vi "Process.vi"(8 "error in":errorcluster, 11 "Inst UI.AH2500":refnum<class "Inst UI.AH2500.lvclass">) -> (0 "error out":errorcluster, 3 "Inst UI.AH2500 out":refnum<class "Inst UI.AH2500.lvclass">)   [LabVIEW 2019, in "Inst UI.AH2500.lvclass"]
doc: "---------------------------------------------------------------\nJKI State Machine Objects™\nhttp://jki.net/state-machine-objects/\nCopyright (C) 2005-2015, JKI <info@jki.net>\nALL RIGHTS RESERVEDJKI State Machine Objects (SMO) 1.0.0.5\nJKI - JKI\nCopyright (c) 2016, JKI"
uses:
  Inst UI.AH2500.lvclass
  C:/Program Files (x86)/National Instruments/LabVIEW 2019/vi.lib/JKI/JKI SMO/SMO/SMO.lvclass
  C:/Program Files (x86)/National Instruments/LabVIEW 2019/user.lib/LevyLab/Instrument Framework/SMOs/Instrument UI/Instrument UI.lvclass
  C:/Program Files (x86)/National Instruments/LabVIEW 2019/vi.lib/JKI/JKI SMO/SMO.UI/SMO.UI.lvclass
  Inst.AH2500/Typedefs/Inst.AH2500.getAll--Cluster.ctl
  Inst.AH2500/Inst.AH2500.lvclass
  C:/Program Files (x86)/National Instruments/LabVIEW 2019/user.lib/LevyLab/Instrument Framework/SMOs/Instrument/Instrument.lvclass
  Inst UI.AH2500.UI--Cluster.ctl
  Inst.AH2500/Typedefs/Inst.AH2500.Configuration--Cluster.ctl
  <userlib>/LevyLab/Instrument Framework/SMOs/Configuration/Configuration.lvclass
  <userlib>/LevyLab/Instrument Framework/SMOs/RemoteControl/Typedefs/Message--Cluster.ctl
  <userlib>/LevyLab/Instrument Framework/SMOs/Instrument UI/Instrument UI.lvclass/Instrument UI.ctl
  Inst.AH2500/Inst.AH2500.lvclass/Inst.AH2500.ctl
  <vilib>/JKI/JKI SMO/SMO/SMO.lvclass/SMO.ctl
  <userlib>/LevyLab/Instrument Framework/SMOs/Configuration/Configuration.lvclass/Configuration.ctl
  <userlib>/LevyLab/Instrument Framework/SMOs/Instrument/Instrument.lvclass/Instrument.ctl
  <userlib>/LevyLab/Instrument Framework/SMOs/Instrument/Typedefs/Client Type--Enum.ctl
  09e9697b-516c-49fb-b2dc-692589121b6f.vi
  <vilib>/JKI/JKI SMO/SMO/Private/ReftoDVR--SMO.vi
  09e9697b-516c-49fb-b2dc-692589121b6f.vi/e95de145-570b-4452-909a-60166876b235.vi
  09e9697b-516c-49fb-b2dc-692589121b6f.vi/e95de145-570b-4452-909a-60166876b235.vi/36141e6f-c45c-4e10-a95a-9d5fe44f6ec9.vi
  <userlib>/LevyLab/Instrument Framework/SMOs/Instrument/API/Send and Receive.vi
  09e9697b-516c-49fb-b2dc-692589121b6f.vi/e95de145-570b-4452-909a-60166876b235.vi/d03f3c8e-ad6b-4901-9eeb-1b6090619d7a.vi
  <userlib>/LevyLab/Instrument Framework/SMOs/Instrument/Private/Get Client Type.vi
  09e9697b-516c-49fb-b2dc-692589121b6f.vi/e95de145-570b-4452-909a-60166876b235.vi/36141e6f-c45c-4e10-a95a-9d5fe44f6ec9.vi/1de991dd-cae7-4693-a0cb-9204aa9fd824.vi
  09e9697b-516c-49fb-b2dc-692589121b6f.vi/e95de145-570b-4452-909a-60166876b235.vi/36141e6f-c45c-4e10-a95a-9d5fe44f6ec9.vi/fe17b767-a917-482f-9198-46e18cb5e30b.vi
  09e9697b-516c-49fb-b2dc-692589121b6f.vi/e95de145-570b-4452-909a-60166876b235.vi/d03f3c8e-ad6b-4901-9eeb-1b6090619d7a.vi/65f50c0c-55d1-4f0e-9c2f-0837c701ede4.vi
  09e9697b-516c-49fb-b2dc-692589121b6f.vi/e95de145-570b-4452-909a-60166876b235.vi/d03f3c8e-ad6b-4901-9eeb-1b6090619d7a.vi/7c5fe90f-b0b4-4563-867a-64d0d40b5a7e.vi
  09e9697b-516c-49fb-b2dc-692589121b6f.vi/e95de145-570b-4452-909a-60166876b235.vi/d03f3c8e-ad6b-4901-9eeb-1b6090619d7a.vi/65f50c0c-55d1-4f0e-9c2f-0837c701ede4.vi/ad86d9d7-fa14-4d0e-9eae-53db6c5c549a.vi
  09e9697b-516c-49fb-b2dc-692589121b6f.vi/e95de145-570b-4452-909a-60166876b235.vi/d03f3c8e-ad6b-4901-9eeb-1b6090619d7a.vi/65f50c0c-55d1-4f0e-9c2f-0837c701ede4.vi/f29f3462-655b-41ba-8fda-c1e4ae9d02a0.vi
  <userlib>/LevyLab/Instrument Framework/SMOs/Instrument/Private/Get RC Connection Status.vi
  <userlib>/LevyLab/Instrument Framework/SMOs/Instrument/API/Enum to String.vi
  <userlib>/LevyLab/Instrument Framework/SMOs/RemoteControl/API/Send and Receive.vi
  <vilib>/Utility/Data Type/Get Type Information.vi
  <vilib>/JDP Science/JSONtext/JSON text to Variant.vi
  <vilib>/JDP Science/JSONtext/Variant to JSON Text.vi
  <vilib>/National Instruments/GUID Generator/Guid Generator.vi
  <userlib>/LevyLab/Instrument Framework/SMOs/Instrument/Private/Instrument.MessageFromProcess.EventStructure.vi
  <userlib>/LevyLab/Instrument Framework/SMOs/Instrument/Instrument.lvclass
  <vilib>/JDP Science/JSONtext/LVClass Serializer/JSONtext LVClass Serializer.lvclass
  <userlib>/LevyLab/Instrument Framework/SMOs/Instrument UI/Instrument UI.lvclass
  <vilib>/JKI/JKI SMO/SMO/SMO.lvclass
  <vilib>/JKI/JKI SMO/SMO.UI/SMO.UI.lvclass
  <userlib>/LevyLab/Instrument Framework/SMOs/RemoteControl/RemoteControl.lvclass
panel:
  in  "Enable Output 2":bool
  in  "I/O":bool
  out "STUFF":bool
  out "LOSS":string="bridge"
  out "CAPACITANCE - pF":string="cap"
  out "Status":string="SMO State: Stopped"
  out "version":string="vDevelopment"
  # "AH 2500A ULTRA-PRECISION 1kHz CAPACITANCE BRIDGE"
  # "SMO UI Template"
  # "For instructions on how to use the JKI State Machine Objects, examples and video tutorials, visit:\nhttp://jki.net/state-machine-objects/\n\nJKI State Machine Objects™\nhttp://jki.net/state-machine-objects/\nCopyright (C) 2005-2015, JKI <info@jki.net>\nALL RIGHTS RESERVED"
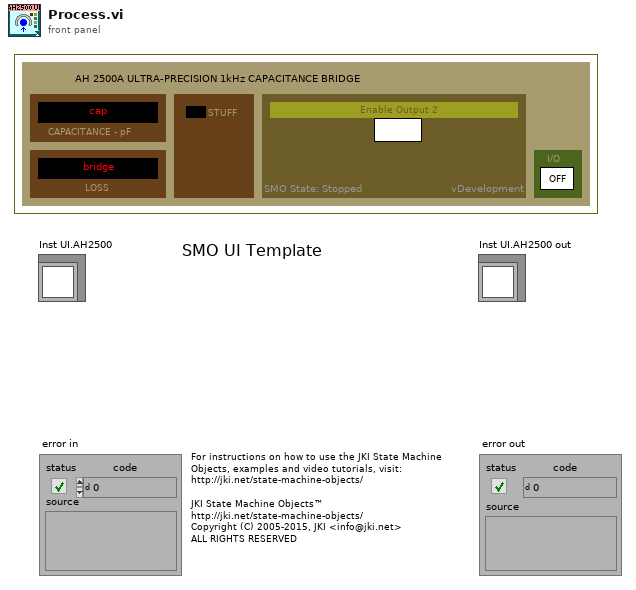
[diagram p1: front panel]
types:
  T1 = enum32{"invalid app kind", "Development System", "Run Time System", "Student Edition", "Embedded LabVIEW", "Evaluation", "Custom"}
  T2 = enum32{"Invalid", "Standard", "Closed", "Hidden", "Minimized", "Maximized"}
  T3 = typedef "Instrument.lvclass/Client Type--Enum.ctl" = enum16{"Remote", "Local"}
  T4 = typedef "RemoteControl.lvclass/Message--Cluster.ctl" = cluster{"Command":string, "Data":variant, "ID":string}
  T5 = typedef "Inst.AH2500.lvclass/Inst.AH2500.Configuration--Cluster.ctl" = cluster{"Example Setting 1":dbl, "Example Setting 2":dbl, "Example Setting 3":string}
  T6 = typedef "Inst.AH2500.lvclass/Inst.AH2500.getAll--Cluster.ctl" = cluster{"capacitance (pF)":dbl, "loss (nS)":dbl, "Vexc (V)":dbl}
  T7 = typedef "Inst UI.AH2500.lvclass/Inst UI.AH2500.UI--Cluster.ctl" = cluster{"Ch1 (V)":dbl, "Ch2 (V)":dbl, "Slew (V/s)":dbl}
  T8 = cluster{"Core":cluster{"Current VI Reference":refnum<vi>, "Close Panel on Exit?":bool, "Last Error":cluster{"error":errorcluster, "previous state":string, "remaining states":string}, "Shutdown?":bool}, "Instrument UI":refnum<class "Inst UI.AH2500.lvclass">, "Instrument":refnum<class "Inst.AH2500.lvclass">, "Configuration":refnum<class "Configuration.lvclass">, "Config Cluster":T5, "getAll":T6, "UI Cluster":T7, "Message":T4}
  T9 = typedef "SMO.lvclass/SMOState --Enum.ctl" = enum16{"unknown", "Created", "Started", "Stopped"}
  T10 = cluster{"Current VI Reference":refnum<vi>, "Close Panel on Exit?":bool, "Last Error":cluster{"error":errorcluster, "previous state":string, "remaining states":string}, "Shutdown?":bool}
  T11 = typedef "SMO.lvclass/Protected Events.ctl" = cluster{"StopProcesses":refnum<user-event>, "AbortProcesses":refnum<user-event>, "Config Changed":refnum<user-event>, "Dependency":refnum<user-event>}
  T12 = typedef "Instrument.lvclass/PublicEvents--Cluster.ctl" = cluster{"MessageFromProcess":refnum<user-event>}
  T13 = typedef "Inst.AH2500.lvclass/PublicEvents--Cluster.ctl" = cluster{"MessageFromProcess":refnum<user-event>}
  T14 = typedef "SMO.lvclass/Public Events.ctl" = cluster{"Error":refnum<user-event>, "State":refnum<user-event>, "Reserve State":refnum<user-event>}
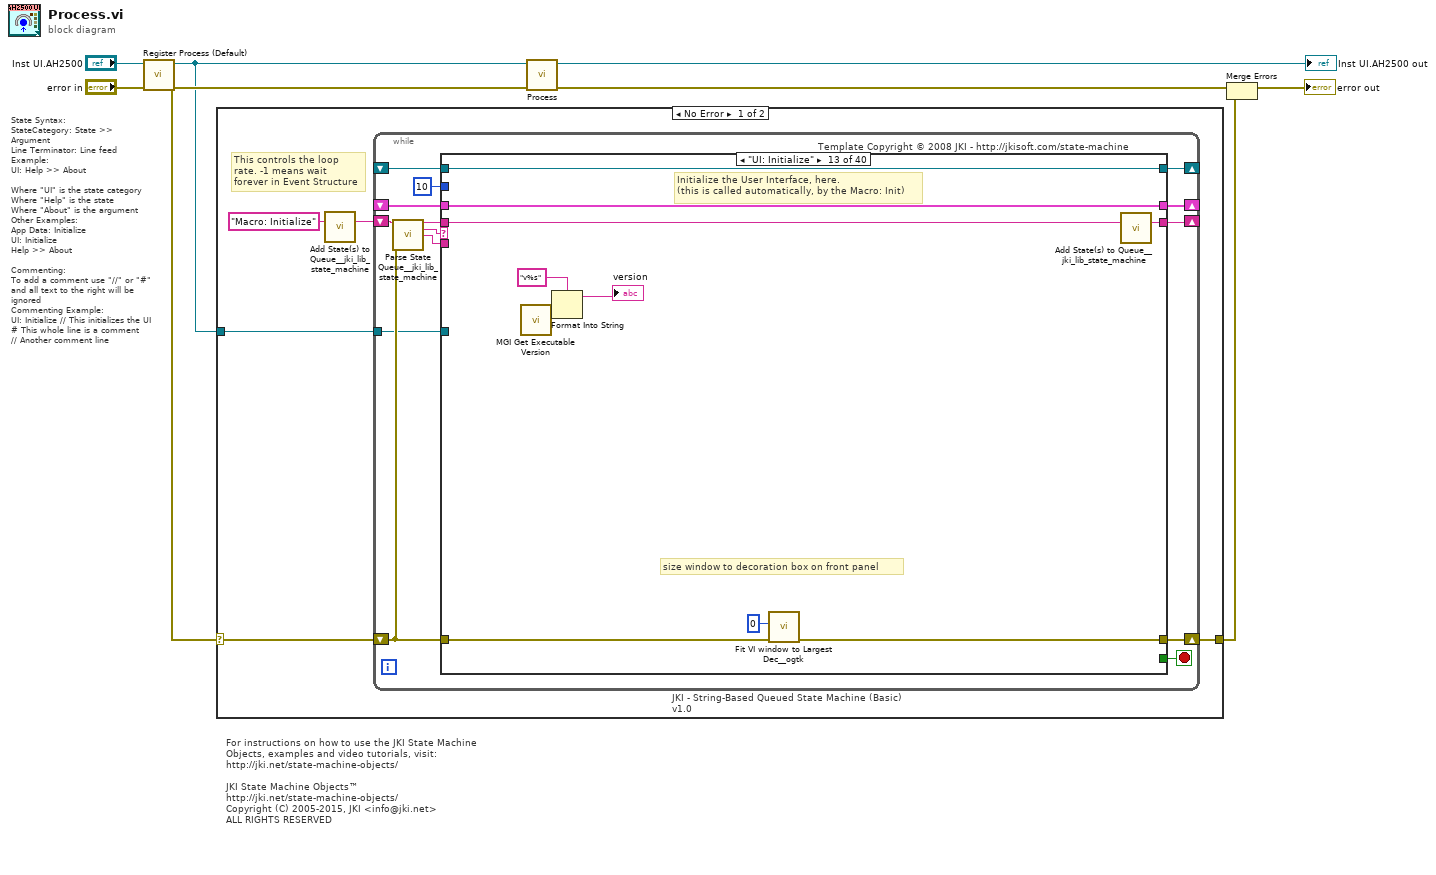
[diagram p0: block diagram]
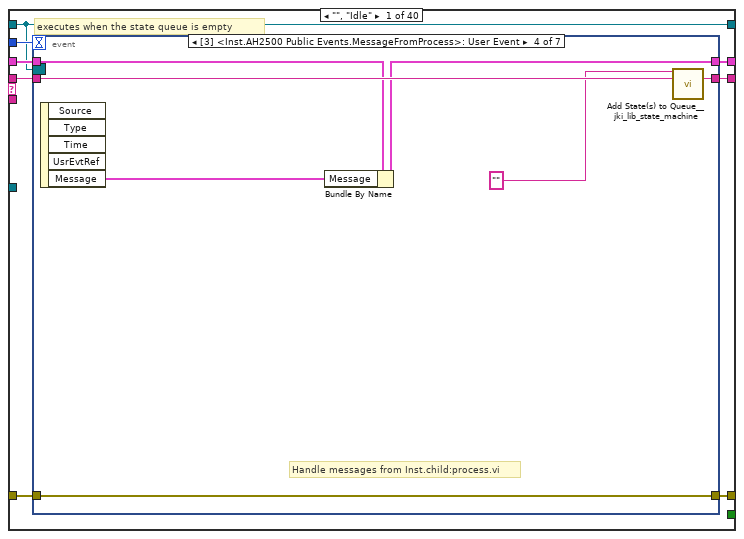
[diagram p2: hidden frame]
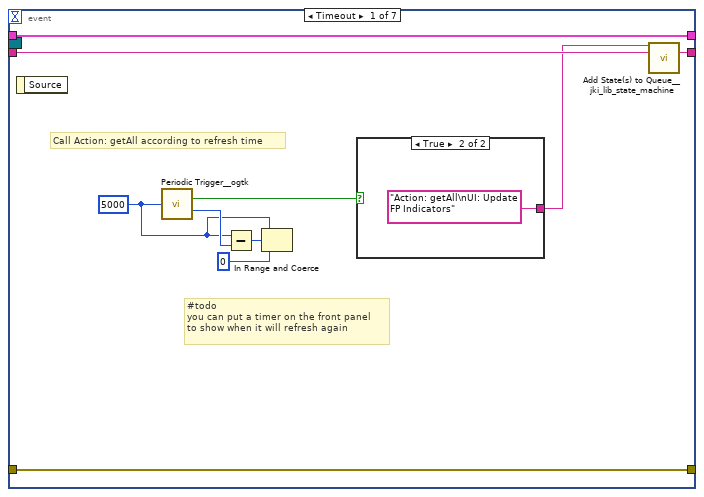
[diagram p3: hidden frame]
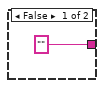
[diagram p4: hidden frame]
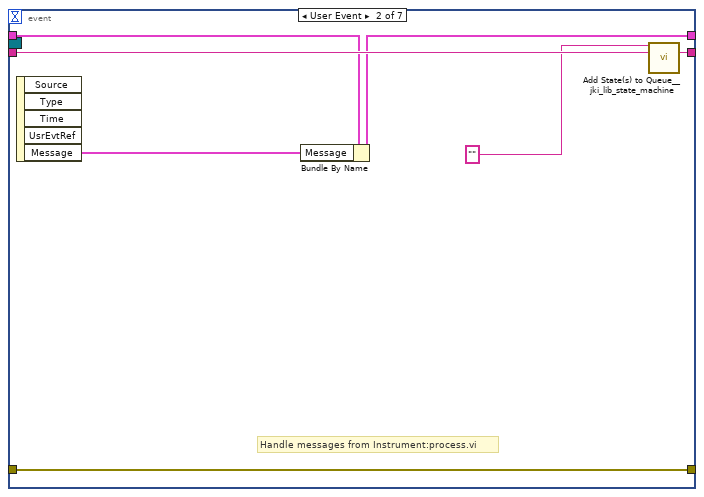
[diagram p5: hidden frame]
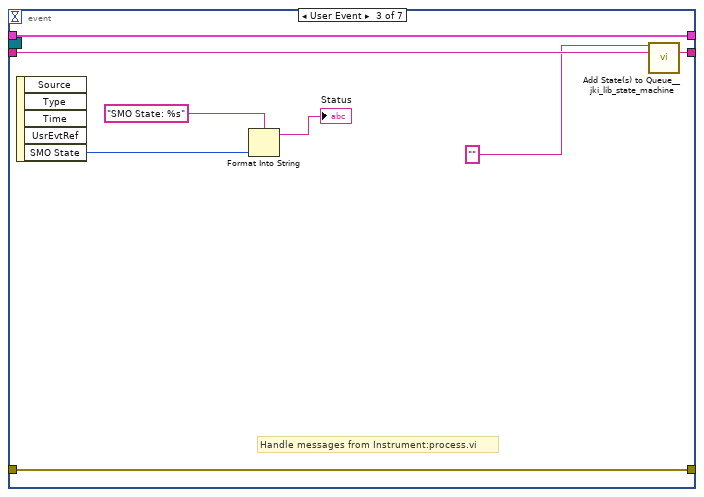
[diagram p6: hidden frame]
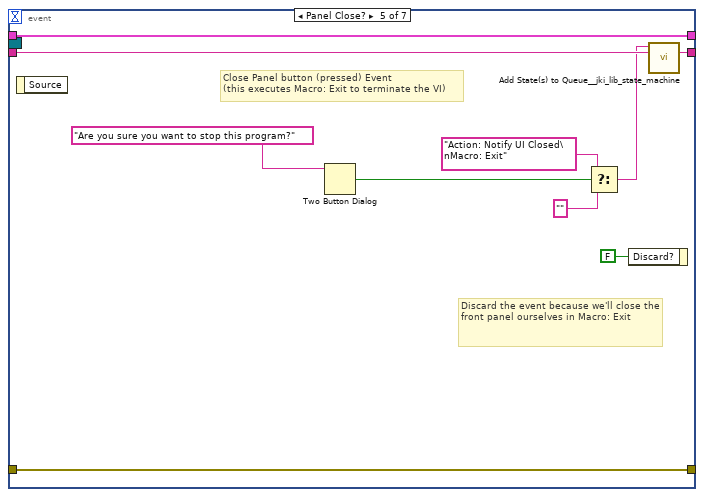
[diagram p7: hidden frame]
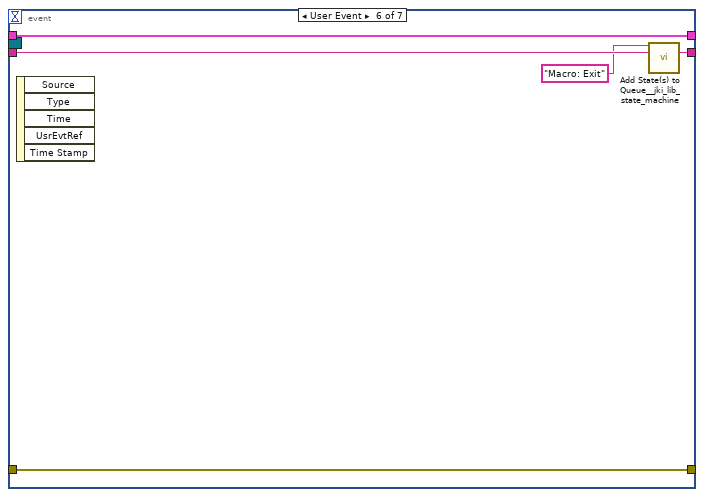
[diagram p8: hidden frame]
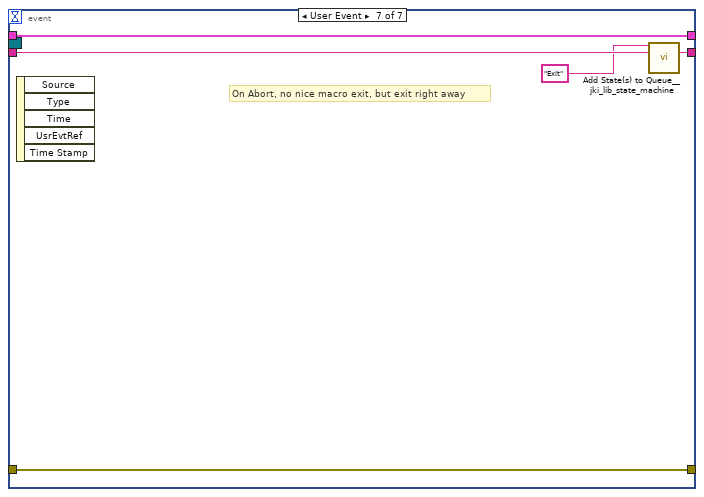
[diagram p9: hidden frame]
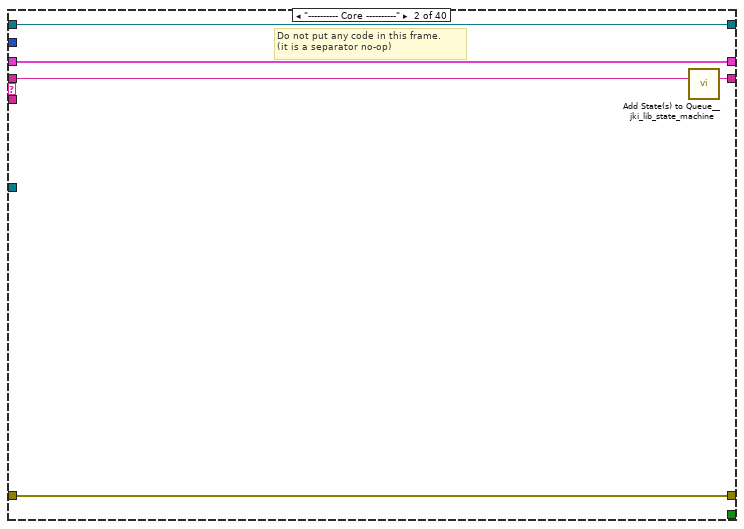
[diagram p10: hidden frame]
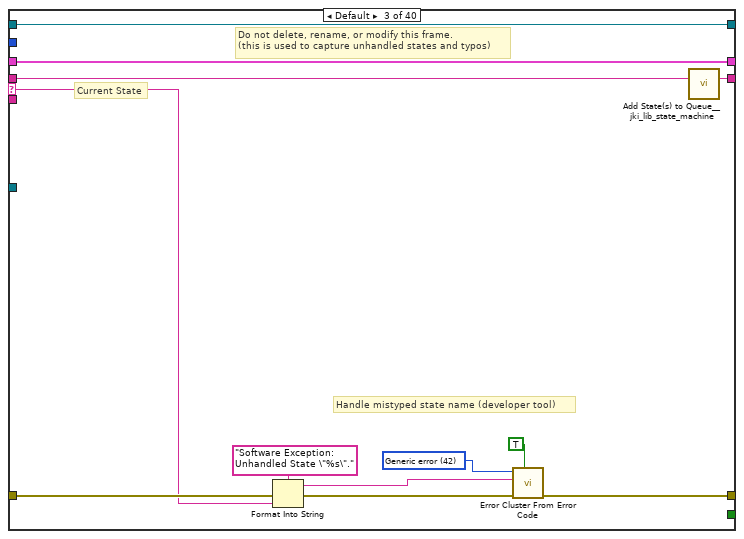
[diagram p11: hidden frame]
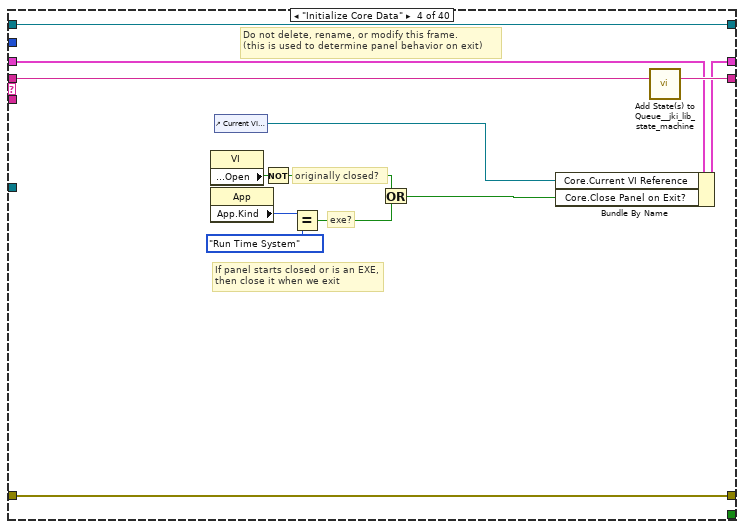
[diagram p12: hidden frame]
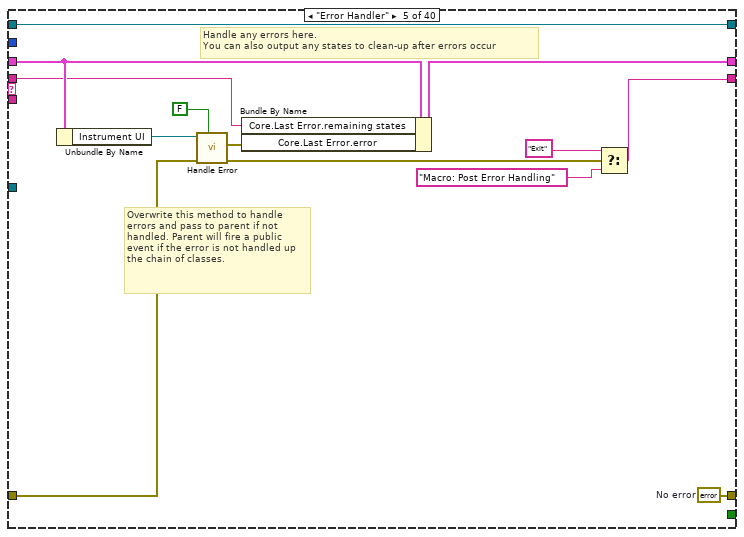
[diagram p13: hidden frame]
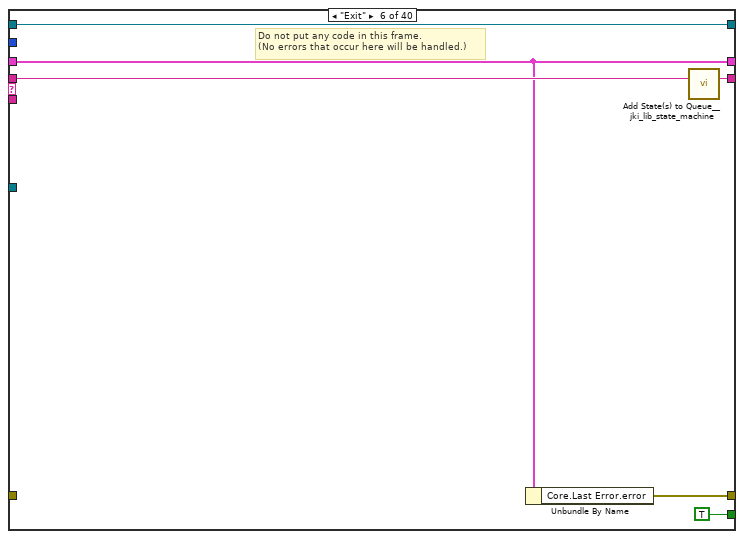
[diagram p14: hidden frame]
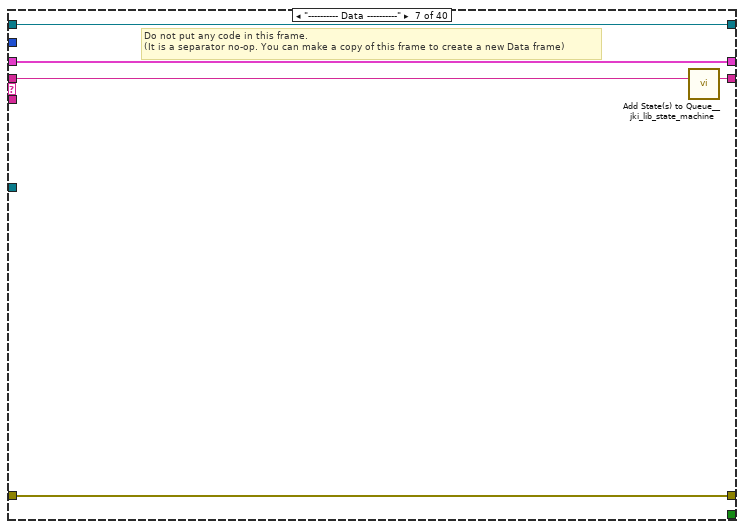
[diagram p15: hidden frame]
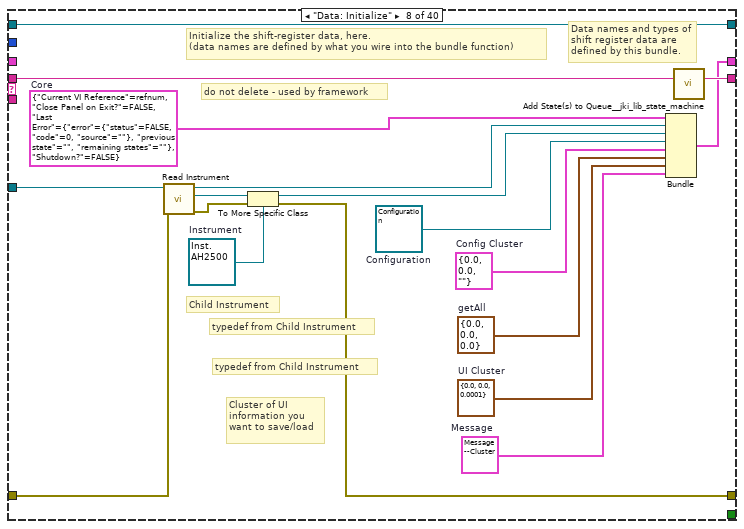
[diagram p16: hidden frame]
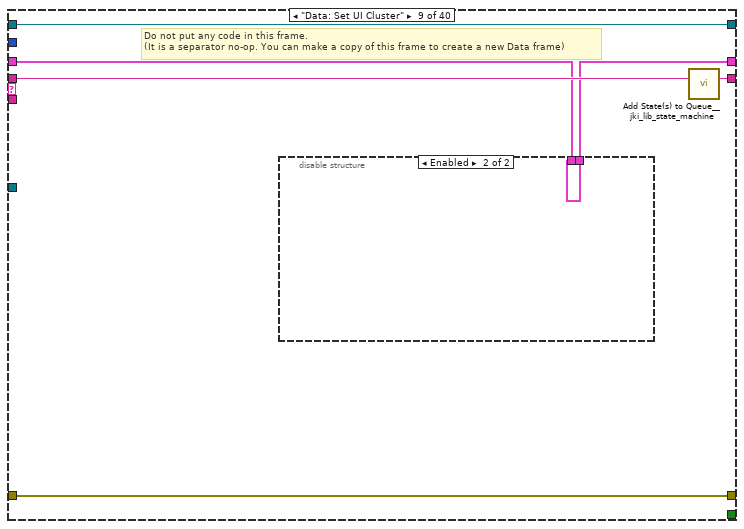
[diagram p17: hidden frame]
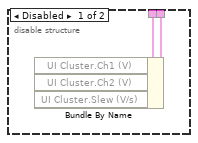
[diagram p18: hidden frame]
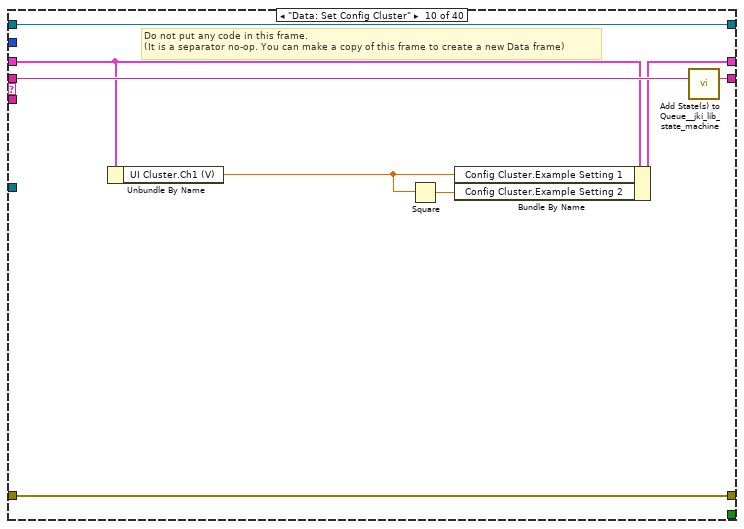
[diagram p19: hidden frame]
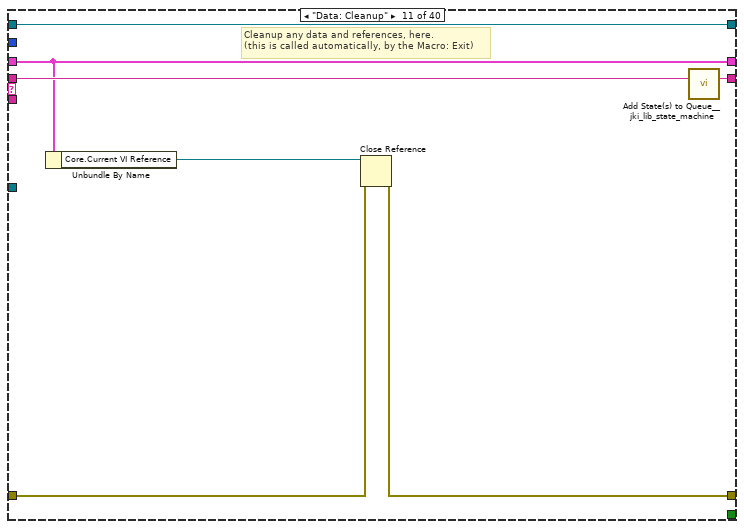
[diagram p20: hidden frame]
diagram:
  # "State Syntax:\nStateCategory: State >> Argument\nLine Terminator: Line feed\nExample:\nUI: Help >> About\n\nWhere \"UI\" is the state category\nWhere \"Help\" is the state\nWhere \"About\" is the argument\nOther Examples:\nApp Data: Initialize\nUI: Initialize\nHelp >> About\n\nCommenting:\nTo add a comment use \"//\" or \"#\" and all text to the right will be ignored\nCommenting Example:\nUI: Initialize // This initializes the UI\n# This whole line is a comment\n// Another comment line"
  # "For instructions on how to use the JKI State Machine Objects, examples and video tutorials, visit:\nhttp://jki.net/state-machine-objects/\n\nJKI State Machine Objects™\nhttp://jki.net/state-machine-objects/\nCopyright (C) 2005-2015, JKI <info@jki.net>\nALL RIGHTS RESERVED"
  n1 = call <vilib>:"Register Process (Default).vi"("error in (no error)"="error in", "SMO"="Inst UI.AH2500") -> ("error out"=w5:errorcluster, "SelfRef"=w4:refnum<class "Inst UI.AH2500.lvclass">)  [unwired: 8 in]
  n2 = case shown="No Error" w5 {
    selector: w5 -> [w10 w487]
    tunnel: w4 -> [w11 _]
    tunnel: [w9 w487] -> w1
    frame No Error {
      # "This controls the loop rate. -1 means wait forever in Event Structure"
      n3 = call <vilib>:"Add State(s) to Queue__jki_lib_state_machine.vi"("State(s) in (\"\")"="Macro: Initialize") -> ("States Out"=w13:string)  [unwired: 14 in]
      n4 = while "JKI - String-Based Queued State Machine (Basic) v1.0" {
        shift-right: [w20] -> _
        shift-left: _ -> [w19]
        shift-right: [w23] -> w9
        shift-left: w10 -> [w17]
        shift-right: [w22] -> _
        shift-left: w13 -> [w24]
        tunnel: w11 -> [w16]
        shift-right: [w15] -> _
        shift-left: _ -> [w14]
        stop <- w21 stop-if-true
        # "Template Copyright © 2008 JKI - http://jkisoft.com/state-machine"
        n5 = call <vilib>:"Parse State Queue__jki_lib_state_machine.vi"("State Queue"=w24, "Error In (no error)"=w17) -> ("Remaining States"=w26:string, "Current State"=w27:string, "Arguments"=w25:string)  [unwired: 11 in]
        n6 = case shown="\"UI: Initialize\"" w27 {
          selector: w27 -> [_ _ w96 _ _ _ _ _ _ _ _ _ _ _ _ _ _ _ _ _ _ _ _ _ _ _ _ _ _ _ _ _ _ _ _ _ _ _ _ _]
          tunnel: w26 -> [w35 w94 w100 w119 w123 w138 w143 w161 w167 w178 w185 w190 w200 w205 w217 w224 w240 w272 w281 w293 w303 w309 w324 w329 w340 w347 w352 w371 w377 w382 w397 w405 w417 w424 w431 w443 w456 w466 w476 w486]
          tunnel: w25 -> [_ _ _ _ _ _ _ _ _ _ _ _ _ _ _ w218 w234 _ _ _ _ _ _ _ _ _ _ _ _ _ _ _ _ _ _ _ _ _ _ _]
          tunnel: w19 -> [w33 w91 w98 w110 w126 w134 w140 _ w163 w174 w179 w187 w198 w201 w213 w222 w236 w269 w277 w283 w300 w306 w311 w326 w337 w342 w349 w369 w375 w379 w390 w402 w408 w419 w425 w435 w450 w458 w471 w481]
          tunnel: [w32 w92 w102 w116 w128 w133 w141 w148 w165 w176 w181 w188 w195 w203 w214 w219 w237 w270 w279 w291 w301 w307 w322 w327 w331 w343 w350 w366 w372 w380 w383 w400 w409 w421 w426 w440 w453 w463 w467 w477] -> w23
          tunnel: w17 -> [w31 w92 w101 w116 w122 _ w141 w145 w165 w176 w182 w188 w196 w203 w214 w220 w238 w270 w279 w291 w301 w307 w322 w327 w332 w344 w350 w356 w373 w380 w392 w398 w410 w421 w427 w436 w445 w459 w468 w478]
          tunnel: [w34 w93 w99 w118 w120 w137 w142 w160 w166 w177 w184 w189 w199 w204 w216 w223 w239 w271 w280 w292 w302 w308 w323 w328 w339 w346 w351 w370 w376 w381 w396 w404 w416 w423 w430 w442 w455 w465 w475 w485] -> w22
          tunnel: [_ _ _ _ _ TRUE _ _ _ _ _ _ _ _ _ _ _ _ _ _ _ _ _ _ _ _ _ _ _ _ _ _ _ _ _ _ _ _ _ _] -> w21
          tunnel: [w30 w91 w98 w117 w125 w134 w140 w159 w162 w173 w179 w187 w198 w201 w213 w222 w236 w269 w277 w284 w300 w306 w311 w326 w337 w342 w349 w369 w375 w379 w394 w402 w406 w418 w425 w437 w451 w460 w472 w482] -> w20
          tunnel: 10 ("Timeout") -> [w29 _ _ _ _ _ _ _ _ _ _ _ _ _ _ _ _ _ _ _ _ _ _ _ _ _ _ _ _ _ _ _ _ _ _ _ _ _ _ _]
          tunnel: w16 -> [_ _ _ _ _ _ _ w146 _ _ _ _ _ _ _ _ _ _ _ _ _ _ _ _ _ _ _ _ _ _ _ _ _ _ _ _ _ _ _ _]
          tunnel: [w28 w90 w95 w107 w132 w135 w139 w158 w164 w175 w180 w186 w197 w202 w215 w221 w233 w268 w278 w290 w299 w305 w316 w325 w338 w345 w348 w368 w374 w378 w395 w403 w415 w422 w429 w441 w454 w464 w474 w484] -> w15
          tunnel: w14 -> [w28 w90 w95 w107 w132 w135 w139 w158 w164 w175 w180 w186 w197 w202 w215 w221 w233 w268 w278 w290 w299 w305 w316 w325 w338 w345 w348 _ w374 w378 w395 w403 w415 w422 w429 w441 w454 w464 w474 w484]
          frame "", "Idle" {
            # "executes when the state queue is empty"
            n7 = event shown="[3] <Inst.AH2500 Public Events.MessageFromProcess>: User Event" {
              selector: w28 -> [_ _ _ _ _ _ _]
              dyn-events: _ -> [_ _ _ _ _ _ _]
              timeout: w29 -> [_ _ _ _ _ _ _]
              tunnel: w35 -> [w45 w54 w62 w69 w79 w84 w89]
              tunnel: [w44 w53 w61 w68 w78 w83 w88] -> w34
              tunnel: w33 -> [w42 w51 w58 w66 w76 w81 w86]
              tunnel: [w43 w52 w60 w67 w75 w82 w87] -> w32
              tunnel: w31 -> [w43 w52 w60 w67 w75 w82 w87]
              tunnel: [w42 w50 w58 w65 w76 w81 w86] -> w30
              event Timeout {
                w37 = u32 5000 ("time (ms)")
                # "#todo\nyou can put a timer on the front panel\nto show when it will refresh again"
                # "Call Action: getAll according to refresh time"
                n8 = event-data() -> ()  [unwired: 1 in, 1 out]
                n9 = call <userlib>:"Periodic Trigger__ogtk.vi"("time (ms)"=w37) -> ("Triggered"=w40:bool, "timer value"=w39:u32)  [unwired: 12 in, 1 out]
                n10 = Subtract(x=w37, y=w39) -> (x-y=w38:u32)
                n11 = In Range and Coerce(upper limit=w37, x=w38, lower limit=u32 0) -> ()  [unwired: 2 out]
                n12 = case shown="True" w40 {
                  tunnel: ["" ("State(s) in Front (\"\")") "Action: getAll\nUI: Update FP Indicators" ("State(s) in Front (\"\")")] -> w41
                  frame False {
                  }
                  frame True {
                  }
                }
                n13 = call <vilib>:"Add State(s) to Queue__jki_lib_state_machine.vi"("State(s) in Front (\"\")"=w41, "State(s) in (\"\")"=w45) -> ("States Out"=w44:string)  [unwired: 13 in]
              }
              event User Event {
                # "Handle messages from Instrument:process.vi"
                n14 = event-data() -> ("Message"=w48:T4)  [unwired: 1 in, 4 out]
                n15 = Bundle By Name(cluster=w51, "Message"=w48) -> (w50:T8)
                n16 = call <vilib>:"Add State(s) to Queue__jki_lib_state_machine.vi"("State(s) in Front (\"\")"="" ("State(s) in Front (\"\")"), "State(s) in (\"\")"=w54) -> ("States Out"=w53:string)  [unwired: 13 in]
              }
              event User Event {
                # "Handle messages from Instrument:process.vi"
                n17 = event-data() -> ("SMO State"=w56:T9)  [unwired: 1 in, 4 out]
                n18 = Format Into String(format string="SMO State: %s", w56) -> (resulting string=→"Status":string)  [unwired: 2 in, 1 out]
                n19 = call <vilib>:"Add State(s) to Queue__jki_lib_state_machine.vi"("State(s) in Front (\"\")"="" ("State(s) in Front (\"\")"), "State(s) in (\"\")"=w62) -> ("States Out"=w61:string)  [unwired: 13 in]
              }
              event User Event {
                # "Handle messages from Inst.child:process.vi"
                n20 = event-data() -> ("Message"=w63:T4)  [unwired: 1 in, 4 out]
                n21 = Bundle By Name(cluster=w66, "Message"=w63) -> (w65:T8)
                n22 = call <vilib>:"Add State(s) to Queue__jki_lib_state_machine.vi"("State(s) in Front (\"\")"="" ("State(s) in Front (\"\")"), "State(s) in (\"\")"=w69) -> ("States Out"=w68:string)  [unwired: 13 in]
              }
              event Panel Close? {
                # "Discard the event because we'll close the front panel ourselves in Macro: Exit"
                # "Close Panel button (pressed) Event\n(this executes Macro: Exit to terminate the VI)"
                n23 = event-data() -> ()  [unwired: 1 in, 1 out]
                n24 = Two Button Dialog(message="Are you sure you want to stop this program?") -> (T button?=w74:bool)  [unwired: 2 in]
                n25 = Select(t="Action: Notify UI Closed\nMacro: Exit", s=w74, f="") -> (s? t:f=w71:string)
                n26 = event-data("Discard?"=FALSE) -> ()  [unwired: 1 in, 1 out]
                n27 = call <vilib>:"Add State(s) to Queue__jki_lib_state_machine.vi"("State(s) in Front (\"\")"=w71, "State(s) in (\"\")"=w79) -> ("States Out"=w78:string)  [unwired: 13 in]
              }
              event User Event {
                n28 = event-data() -> ()  [unwired: 1 in, 5 out]
                n29 = call <vilib>:"Add State(s) to Queue__jki_lib_state_machine.vi"("State(s) in Front (\"\")"="Macro: Exit", "State(s) in (\"\")"=w84) -> ("States Out"=w83:string)  [unwired: 13 in]
              }
              event User Event {
                # "On Abort, no nice macro exit, but exit right away"
                n30 = event-data() -> ()  [unwired: 1 in, 5 out]
                n31 = call <vilib>:"Add State(s) to Queue__jki_lib_state_machine.vi"("State(s) in Front (\"\")"="Exit", "State(s) in (\"\")"=w89) -> ("States Out"=w88:string)  [unwired: 13 in]
              }
            }
          }
          frame "---------- Core ----------" {
            # "Do not put any code in this frame.\n(it is a separator no-op)"
            n32 = call <vilib>:"Add State(s) to Queue__jki_lib_state_machine.vi"("State(s) in (\"\")"=w94) -> ("States Out"=w93:string)  [unwired: 14 in]
          }
          frame Default {
            w105 = 42 items=["No error", "Argument error", "Memory is full", "Out of zone", "End of file", "File already open", "Generic file I/O error", "File not found", "File permission error", "Disk is full", "Duplicate path", "Too many files open", "System feature not enabled", "Resource file not found", "Cannot add resource", "Resource not found", "Image not found", "Image memory error", "Pen does not exist", "Config type invalid", "Config token not found", "Config parse error", "Config memory error", "Bad external code format", "Bad external code offset", "External code not present", "Null window", "Destroy window error", "Null menu", "Print aborted", "Bad print record", "Print driver error", "Windows error during printing", "Memory error during printing", "Print dialog error", "Generic print error", "Invalid device refnum", "Device not found", "Device parameter error", "Device unit error", "Cannot open device", "Device call aborted", "Generic error", "Cancelled by user", "Object ID too low", "Object ID too high", "Object not in heap", "Unknown heap", "Unknown object (invalid DefProc)", "Unknown object (DefProc not in table)", "Message out of range", "Invalid (null) method", "Unknown message", "Manager call not supported", "Bad address", "Network operation in progress", "Network operation timed out", "Connection is busy", "Network attribute not supported", "Network error", "Address in use", "System out of memory", "Connection aborted", "Connection refused", "Not connected", "Already connected", "Connection closed", "Initialization error (interapplication manager)", "Bad occurrence", "Wait on unbound occurrence handler", "Occurrence queue overflow", "Datalog type conflict", "Unused", "Unrecognized type (interapplication manager)", "Memory corrupt", "Failed to make temporary DLL", "Old CIN version", "Drag socket not found", "Failed to load drop-object", "Failed to register OLE object", "Failed to release OLE object", "Format specifier type mismatch", "Unknown format specifier", "Too few format specifiers", "Too many format specifiers", "Scan failed", "Newer CIN version", "Error converting to variant", "Runtime menu error", "Password tampered", "Variant attribute not found", "Incompatible variant data type", "Event data is not available", "Event Store is not present", "Occurrence is not found", "Event Queue is not created", "Event info is not available", "Refnum passed is NULL", "Error retrieving Class GUID", "Error retrieving CoClass GUID", "Error retrieving TypeLib GUID.", "Bad built application magic bytes.", "Specific driver is different from the specific driver associated with the Logical Name.", "There is no session opened to the class driver.", "Max Error", "MAX - Error with config objects", "MAX - Error loading configuration", "MAX - Group not supported"]
            # "Current State"
            # "Do not delete, rename, or modify this frame.\n(this is used to capture unhandled states and typos)"
            # "Handle mistyped state name (developer tool)"
            n33 = Format Into String(format string="Software Exception: Unhandled State \"%s\"." ("message"), error in=w101, w96) -> (resulting string=w104:string, error out=w103:errorcluster)  [unwired: 1 in]
            n34 = call <vilib>:"Error Cluster From Error Code.vi"("show call chain? (False)"=TRUE, "error in (no error)"=w103, "error message (\"\")"=w104, "error code (0)"=w105) -> ("error out"=w102:errorcluster)  [unwired: 5 in]
            n35 = call <vilib>:"Add State(s) to Queue__jki_lib_state_machine.vi"("State(s) in (\"\")"=w100) -> ("States Out"=w99:string)  [unwired: 14 in]
          }
          frame "Initialize Core Data" {
            # "Do not delete, rename, or modify this frame.\n(this is used to determine panel behavior on exit)"
            # "originally closed?"
            # "exe?"
            # "If panel starts closed or is an EXE, then close it when we exit"
            n36 = property class="VI"() -> ("Front Panel.Open"=w115:bool)  [unwired: 2 in, 2 out]
            n37 = property class="App"() -> ("App.Kind"=w114:T1)  [unwired: 2 in, 2 out]
            n38 = control-ref of="Current VI Reference"() -> (w108:refnum<vi>)
            n39 = Not(x=w115) -> (.not. x?=w112:bool)
            n40 = Equal?(x=w114, y=T1."Run Time System" ("Application:Kind")) -> (x = y?=w111:bool)
            n41 = Or(x=w112, y=w111) -> (x .or. y?=w109:bool)
            n42 = Bundle By Name(cluster=w110, "Core.Current VI Reference"=w108, "Core.Close Panel on Exit?"=w109) -> (w117:T8)
            n43 = call <vilib>:"Add State(s) to Queue__jki_lib_state_machine.vi"("State(s) in (\"\")"=w119) -> ("States Out"=w118:string)  [unwired: 14 in]
          }
          frame "Error Handler" {
            w128 = errorcluster {"status"=FALSE, "code"=0, "source"=""}  # No error
            # "Overwrite this method to handle errors and pass to parent if not handled. Parent will fire a public event if the error is not handled up the chain of classes."
            # "Handle any errors here.\nYou can also output any states to clean-up after errors occur"
            n44 = Unbundle By Name(w126) -> ("Instrument UI"=w131:refnum<class "Inst UI.AH2500.lvclass">)
            n45 = call-dynamic "Handle Error.vi"("Stop on Unhandled Error (T)"=FALSE, "error in"=w122, "SMO"=w131) -> ("handling error"=w129:errorcluster, "Unhandled error"=w127:errorcluster)  [unwired: 6 in, 1 out]
            n46 = Bundle By Name(cluster=w126, "Core.Last Error.remaining states"=w123, "Core.Last Error.error"=w127) -> (w125:T8)
            n47 = Select(t="Exit", s=w129, f="Macro: Post Error Handling") -> (s? t:f=w120:string)
          }
          frame "Exit" {
            # "Do not put any code in this frame.\n(No errors that occur here will be handled.)"
            n48 = Unbundle By Name(w134) -> ("Core.Last Error.error"=w133:errorcluster)
            n49 = call <vilib>:"Add State(s) to Queue__jki_lib_state_machine.vi"("State(s) in (\"\")"=w138) -> ("States Out"=w137:string)  [unwired: 14 in]
          }
          frame "---------- Data ----------" {
            # "Do not put any code in this frame.\n(It is a separator no-op. You can make a copy of this frame to create a new Data frame)"
            n50 = call <vilib>:"Add State(s) to Queue__jki_lib_state_machine.vi"("State(s) in (\"\")"=w143) -> ("States Out"=w142:string)  [unwired: 14 in]
          }
          frame "Data: Initialize" {
            w144 = T4 {"Command"="", "Data"=variant, "ID"=""}  # Message
            w147 = refnum<class "Configuration.lvclass"> refnum  # Configuration
            w150 = T5 {"Example Setting 1"=0.0, "Example Setting 2"=0.0, "Example Setting 3"=""}  # Config Cluster
            w152 = T7 {"Ch1 (V)"=0.0, "Ch2 (V)"=0.0, "Slew (V/s)"=0.0001}  # UI Cluster
            w154 = refnum<class "Inst.AH2500.lvclass"> refnum  # Instrument
            w156 = T6 {"capacitance (pF)"=0.0, "loss (nS)"=0.0, "Vexc (V)"=0.0}  # getAll
            w157 = T10 {"Current VI Reference"=refnum, "Close Panel on Exit?"=FALSE, "Last Error"={"error"={"status"=FALSE, "code"=0, "source"=""}, "previous state"="", "remaining states"=""}, "Shutdown?"=FALSE}  # Core
            # "typedef from Child Instrument"
            # "Cluster of UI\ninformation you\nwant to save/load"
            # "Child Instrument"
            # "typedef from Child Instrument"
            # "do not delete - used by framework"
            # "Data names and types of shift register data are defined by this bundle."
            # "Initialize the shift-register data, here.\n(data names are defined by what you wire into the bundle function)"
            n51 = call <userlib>:"Read Instrument.vi"("error in (no error)"=w145, "Instrument UI in"=w146) -> ("error out"=w151:errorcluster, "Instrument"=w153:refnum<class "Instrument.lvclass">, "Instrument UI"=w155:refnum<class "Inst UI.AH2500.lvclass">)  [unwired: 7 in]
            n52 = To More Specific Class(target class=w154, reference=w153, error in=w151) -> (specific class reference=w149:refnum<class "Inst.AH2500.lvclass">, error out=w148:errorcluster)
            n53 = Bundle("Core"=w157, "Instrument UI"=w155, "Instrument"=w149, "Configuration"=w147, "Config Cluster"=w150, "getAll"=w156, "UI Cluster"=w152, "Message"=w144) -> (w159:T8)  [unwired: 1 in]
            n54 = call <vilib>:"Add State(s) to Queue__jki_lib_state_machine.vi"("State(s) in (\"\")"=w161) -> ("States Out"=w160:string)  [unwired: 14 in]
          }
          frame "Data: Set UI Cluster" {
            # "Do not put any code in this frame.\n(It is a separator no-op. You can make a copy of this frame to create a new Data frame)"
            n55 = disable-structure shown="Enabled" {
              disable-tunnel: w163 -> [w169 w170]
              disable-tunnel: [w168 w170] -> w162
              frame Disabled {
                n56 = Bundle By Name(cluster=w169) -> (w168:T8)  [unwired: 3 in]
              }
              frame Enabled {
              }
            }
            n57 = call <vilib>:"Add State(s) to Queue__jki_lib_state_machine.vi"("State(s) in (\"\")"=w167) -> ("States Out"=w166:string)  [unwired: 14 in]
          }
          frame "Data: Set Config Cluster" {
            # "Do not put any code in this frame.\n(It is a separator no-op. You can make a copy of this frame to create a new Data frame)"
            n58 = Unbundle By Name(w174) -> ("UI Cluster.Ch1 (V)"=w172:dbl)
            n59 = Square(x=w172) -> (x^2=w171:dbl)
            n60 = Bundle By Name(cluster=w174, "Config Cluster.Example Setting 1"=w172, "Config Cluster.Example Setting 2"=w171) -> (w173:T8)
            n61 = call <vilib>:"Add State(s) to Queue__jki_lib_state_machine.vi"("State(s) in (\"\")"=w178) -> ("States Out"=w177:string)  [unwired: 14 in]
          }
          frame "Data: Cleanup" {
            # "Cleanup any data and references, here.\n(this is called automatically, by the Macro: Exit)"
            n62 = Unbundle By Name(w179) -> ("Core.Current VI Reference"=w183:refnum<vi>)
            n63 = Close Reference(reference=w183, error in (no error)=w182) -> (error out=w181:errorcluster)
            n64 = call <vilib>:"Add State(s) to Queue__jki_lib_state_machine.vi"("State(s) in (\"\")"=w185) -> ("States Out"=w184:string)  [unwired: 14 in]
          }
          frame "---------- UI ----------" {
            # "Do not put any code in this frame.\n(It is a separator no-op. You can make a copy of this frame to create a new UI frame)"
            n65 = call <vilib>:"Add State(s) to Queue__jki_lib_state_machine.vi"("State(s) in (\"\")"=w190) -> ("States Out"=w189:string)  [unwired: 14 in]
          }
          frame "UI: Initialize" {
            # "size window to decoration box on front panel"
            # "Initialize the User Interface, here.\n(this is called automatically, by the Macro: Init)"
            n66 = call <userlib>:"MGI Get Executable Version.vi"() -> ("Version"=w193:string)  [unwired: 7 in]
            n67 = Format Into String(format string="v%s", w193) -> (resulting string=→"version":string)  [unwired: 2 in, 1 out]
            n68 = call <userlib>:"Fit VI window to Largest Dec__ogtk.vi"("error in (no error)"=w196, "border spacing (2 px)"=0) -> ("error out"=w195:errorcluster)  [unwired: 4 in, 1 out]
            n69 = call <vilib>:"Add State(s) to Queue__jki_lib_state_machine.vi"("State(s) in (\"\")"=w200) -> ("States Out"=w199:string)  [unwired: 14 in]
          }
          frame "UI: Update FP Controls" {
            # "Do not put any code in this frame.\n(It is a separator no-op. You can make a copy of this frame to create a new UI frame)"
            n70 = Unbundle By Name(w201) -> ()  [unwired: 3 out]
            n71 = call <vilib>:"Add State(s) to Queue__jki_lib_state_machine.vi"("State(s) in (\"\")"=w205) -> ("States Out"=w204:string)  [unwired: 14 in]
          }
          frame "UI: Update FP Indicators" {
            n72 = Unbundle By Name(w213) -> ("getAll"=w212:T6)
            n73 = Unbundle By Name(w212) -> ("capacitance (pF)"=w207:dbl, "loss (nS)"=w206:dbl)
            n74 = Format Into String(format string="%08.7f" ("Status 6"), w206) -> (resulting string=→"LOSS":string)  [unwired: 2 in, 1 out]
            n75 = Format Into String(format string="%08.7f" ("Status 6"), w207) -> (resulting string=→"CAPACITANCE - pF":string)  [unwired: 2 in, 1 out]
            n76 = call <vilib>:"Add State(s) to Queue__jki_lib_state_machine.vi"("State(s) in (\"\")"=w217) -> ("States Out"=w216:string)  [unwired: 14 in]
          }
          frame "UI: Cursor Set" {
            # "Argument"
            # "Initialize the User Interface, here.\n(this is called automatically, by the Macro: Init)"
            n77 = disable-structure shown="Default" {
              disable-tunnel: w220 -> [w225 w228]
              disable-tunnel: [w225 w227] -> w219
              disable-tunnel: w218 -> [_ w226]
              frame condition #0 {
              }
              frame condition #1 (active) {
                n78 = case shown="\"Busy\"" w226 {
                  tunnel: w228 -> [w230 w232]
                  tunnel: [w229 w231] -> w227
                  frame "Idle", Default {
                    n79 = call <vilib>:"Unset Busy.vi"("error in (no error)"=w230) -> ("error out"=w229:errorcluster)  [unwired: 10 in]
                  }
                  frame "Busy" {
                    n80 = call <vilib>:"Set Busy.vi"("error in (no error)"=w232) -> ("error out"=w231:errorcluster)  [unwired: 9 in, 1 out]
                  }
                }
              }
            }
            n81 = call <vilib>:"Add State(s) to Queue__jki_lib_state_machine.vi"("State(s) in (\"\")"=w224) -> ("States Out"=w223:string)  [unwired: 14 in]
          }
          frame "UI: Front Panel State" {
            # "Argument"
            # "Set Front Panel Open or Closed\n(Usage: \"UI: Front Panel State >> Open|Close\")"
            n82 = Unbundle By Name(w236) -> ("Core.Current VI Reference"=w235:refnum<vi>)
            n83 = disable-structure shown="Default" {
              disable-tunnel: w238 -> [w244 w267]
              disable-tunnel: [w243 w267] -> w237
              disable-tunnel: w235 -> [w242 _]
              disable-tunnel: w234 -> [w241 _]
              frame condition #0 (active) {
                n84 = case shown="\"Close\"" w241 {
                  tunnel: w244 -> [w248 w261]
                  tunnel: [w250 w262] -> w243
                  tunnel: w242 -> [w249 w259]
                  frame "Open", Default {
                    n85 = property class="VI"(reference=w249, error in=w248) -> (reference out=w246:refnum<vi>, error out=w247:errorcluster, "FP.State"=w245:T2)
                    n86 = case shown="\"Closed\"" w245 {
                      tunnel: [w253 w256] -> w250
                      tunnel: w247 -> [w252 w256]
                      tunnel: w246 -> [w251 _]
                      frame "Closed" {
                        n87 = invoke class="VI" method="FP.Open"(reference=w251, error in=w252, "Activate"=TRUE, "State"=T2."Standard") -> (error out=w253:errorcluster)  [unwired: 1 in, 4 out]
                      }
                      frame Default {
                      }
                    }
                  }
                  frame "Close" {
                    n88 = property class="VI"(reference=w259, error in=w261) -> (reference out=w258:refnum<vi>, error out=w260:errorcluster, "FP.State"=w257:T2)
                    n89 = case shown="Default" w257 {
                      tunnel: [w263 w266] -> w262
                      tunnel: w260 -> [w263 w265]
                      tunnel: w258 -> [_ w264]
                      frame "Invalid", "Closed" {
                      }
                      frame Default {
                        n90 = invoke class="VI" method="FP.Close"(reference=w264, error in=w265) -> (error out=w266:errorcluster)  [unwired: 1 in, 2 out]
                      }
                    }
                  }
                }
              }
              frame condition #1 {
              }
            }
            n91 = call <vilib>:"Add State(s) to Queue__jki_lib_state_machine.vi"("State(s) in (\"\")"=w240) -> ("States Out"=w239:string)  [unwired: 14 in]
          }
          frame "---------- Macro ----------" {
            # "Do not put any code in this frame.\n(It is a separator no-op. You can make a copy of this frame to create a new Macro frame)"
            n92 = call <vilib>:"Add State(s) to Queue__jki_lib_state_machine.vi"("State(s) in (\"\")"=w272) -> ("States Out"=w271:string)  [unwired: 14 in]
          }
          frame "Macro: Initialize" {
            w275 = "UI: Initialize\nMacro: Read UI Config\nAction: Open\n//UI: Front Panel State >> Open"  # UI: Initialize Macro: Read UI Config Action: Open //UI: Front Panel State >> Open
            # "Initialization Macro\n(This is called once, when the VI starts)"
            n93 = call <vilib>:"Add State(s) to Queue__jki_lib_state_machine.vi"("State(s) in Front (\"\")"="Data: Initialize\nInitialize Core Data\nEvents: Register", "State(s) in (\"\")"="Process: Sync", "State(s) at Back (\"\")"=w275) -> ("States Out"=w274:string)  [unwired: 12 in]
            n94 = call <vilib>:"Add State(s) to Queue__jki_lib_state_machine.vi"("State(s) in Front (\"\")"=w274, "State(s) in (\"\")"=w281) -> ("States Out"=w280:string)  [unwired: 13 in]
          }
          frame "Macro: Post Error Handling" {
            # "Clear Last Error?"
            n95 = Unbundle By Name(w283) -> ("Core.Last Error.remaining states"=w285:string, "Core.Shutdown?"=w286:bool)
            n96 = Unbundle By Name(w283) -> ("Core.Last Error.error"=w289:errorcluster)
            n97 = case shown="False" FALSE {
              tunnel: w289 -> [w297 _]
              tunnel: [w297 _] -> w288
              frame False {
              }
              frame True {
              }
            }
            n98 = case shown="False" w286 {
              tunnel: w285 -> [w294 w296]
              tunnel: [w294 w295] -> w282
              frame False {
                # "These are the remaining states (at the moment the error occured). States can be altered according to business logic."
                # "NOT SHUTTING DOWN"
              }
              frame True {
                # "Developer can decide to alter the states but should be aware that during the shutdown process, there are certain states that must be run for the SMO to properly shut itself (and this process) down. As such, one can add states to perform additional clean-ups, but should append the remaining state to be executed."
                # "SHUTTING DOWN"
                n99 = call <vilib>:"Add State(s) to Queue__jki_lib_state_machine.vi"("State(s) in (\"\")"=w296) -> ("States Out"=w295:string)  [unwired: 14 in]
              }
            }
            n100 = Bundle By Name(cluster=w283, "Core.Last Error.error"=w288) -> (w284:T8)
            n101 = call <vilib>:"Add State(s) to Queue__jki_lib_state_machine.vi"("State(s) in Front (\"\")"=w282, "State(s) in (\"\")"=w293) -> ("States Out"=w292:string)  [unwired: 13 in]
          }
          frame "Macro: Read UI Config" {
            # "Do not put any code in this frame.\n(It is a separator no-op. You can make a copy of this frame to create a new Macro frame)"
            n102 = call <vilib>:"Add State(s) to Queue__jki_lib_state_machine.vi"("State(s) in Front (\"\")"="Configuration: Initialize\nConfiguration: Read UI Config File\nUI: Update FP Controls" ("State(s) in Front (\"\")"), "State(s) in (\"\")"=w303) -> ("States Out"=w302:string)  [unwired: 13 in]
          }
          frame "Macro: Write UI Config" {
            # "Do not put any code in this frame.\n(It is a separator no-op. You can make a copy of this frame to create a new Macro frame)"
            n103 = call <vilib>:"Add State(s) to Queue__jki_lib_state_machine.vi"("State(s) in Front (\"\")"="Data: Set UI Cluster\nConfiguration: Write UI Config File" ("State(s) in Front (\"\")"), "State(s) in (\"\")"=w309) -> ("States Out"=w308:string)  [unwired: 13 in]
          }
          frame "Macro: Exit" {
            # "Exit Macro\n(This is called once, when the VI exits)"
            n104 = Unbundle By Name(w311) -> ("Core.Close Panel on Exit?"=w321:bool)
            n105 = Select(t="UI: Front Panel State >> Close", s=w321, f="" ("Empty String Constant")) -> (s? t:f=w318:string)
            n106 = call <vilib>:"Add State(s) to Queue__jki_lib_state_machine.vi"("State(s) in Front (\"\")"="Data: Cleanup\nEvents: Unregister\nProcess: Self Terminate", "State(s) in (\"\")"="Process: Sync", "State(s) at Back (\"\")"="Exit") -> ("States Out"=w313:string)  [unwired: 12 in]
            n107 = call <vilib>:"Add State(s) to Queue__jki_lib_state_machine.vi"("State(s) in Front (\"\")"="Action: Close\nMacro: Write UI Config", "State(s) in (\"\")"=w318, "State(s) at Back (\"\")"=w313) -> ("States Out"=w317:string)  [unwired: 12 in]
            n108 = call <vilib>:"Add State(s) to Queue__jki_lib_state_machine.vi"("State(s) in Front (\"\")"=w317, "State(s) in (\"\")"=w324) -> ("States Out"=w323:string)  [unwired: 13 in]
          }
          frame "---------- Process ----------" {
            # "Template Separator\n(You can make a copy of, or modify, this frame)"
            n109 = call <vilib>:"Add State(s) to Queue__jki_lib_state_machine.vi"("State(s) in (\"\")"=w329) -> ("States Out"=w328:string)  [unwired: 14 in]
          }
          frame "Process: Sync" {
            n110 = Unbundle By Name(w337) -> ("Instrument UI"=w333:refnum<class "Inst UI.AH2500.lvclass">)
            n111 = call <vilib>:"WaitOnProcessSync.vi"("error in (no error)"=w332, "SMO"=w333) -> ("error out"=w331:errorcluster, "Don't run?"=w336:bool)  [unwired: 7 in, 1 out]
            n112 = Select(t="Data: Cleanup\nEvents: Unregister\nExit", s=w336, f="" ("Empty String Constant")) -> (s? t:f=w330:string)
            n113 = call <vilib>:"Add State(s) to Queue__jki_lib_state_machine.vi"("State(s) in Front (\"\")"=w330, "State(s) in (\"\")"=w340) -> ("States Out"=w339:string)  [unwired: 13 in]
          }
          frame "Process: Self Terminate" {
            n114 = Unbundle By Name(w342) -> ("Instrument UI"=w341:refnum<class "Inst UI.AH2500.lvclass">)
            n115 = call <vilib>:"SelfTerminate.vi"("error in (no error)"=w344, "SMO in"=w341) -> ("error out"=w343:errorcluster)  [unwired: 8 in, 1 out]
            n116 = call <vilib>:"Add State(s) to Queue__jki_lib_state_machine.vi"("State(s) in (\"\")"=w347) -> ("States Out"=w346:string)  [unwired: 14 in]
          }
          frame "---------- Events ----------" {
            # "Template Separator\n(You can make a copy of, or modify, this frame)"
            n117 = call <vilib>:"Add State(s) to Queue__jki_lib_state_machine.vi"("State(s) in (\"\")"=w352) -> ("States Out"=w351:string)  [unwired: 14 in]
          }
          frame "Events: Register" {
            # "Expand to add\nmore events"
            # "Base Class Protected Events"
            n118 = Unbundle By Name(w369) -> ("Instrument UI"=w362:refnum<class "Inst UI.AH2500.lvclass">, "Instrument"=w361:refnum<class "Inst.AH2500.lvclass">)
            n119 = call <vilib>:"GetProtectedEvents.vi"("SMO"=w362) -> ("error out"=w365:errorcluster, "SMO Protected Events"=w367:T11)  [unwired: 8 in, 1 out]
            n120 = call <userlib>:"Instrument.GetPublicEvents.vi"("Instrument"=w361) -> ("error out"=w363:errorcluster, "Instrument Public Events"=w364:T12, "Instrument out"=w359:refnum<class "Inst.AH2500.lvclass">)  [unwired: 8 in]
            n121 = call "Inst.AH2500.GetPublicEvents.vi"("Inst.AH2500 in"=w359) -> ("error out"=w358:errorcluster, "Inst.AH2500 Public Events"=w360:T13, "Inst.AH2500 out"=w355:refnum<class "Inst.AH2500.lvclass">)  [unwired: 8 in]
            n122 = call <vilib>:"GetPublicEvents.vi"("SMO"=w355) -> ("error out"=w353:errorcluster, "Public Events"=w354:T14)  [unwired: 8 in, 1 out]
            n123 = register-events(w367, w364, w360, w354) -> (reference out=w368:refnum<event-registration>, error out=w357:errorcluster)  [unwired: 2 in]
            n124 = Merge Errors(w357, w353, w358, w363, w365, w356) -> (w366:errorcluster)
            n125 = call <vilib>:"Add State(s) to Queue__jki_lib_state_machine.vi"("State(s) in (\"\")"=w371) -> ("States Out"=w370:string)  [unwired: 14 in]
          }
          frame "Events: Unregister" {
            n126 = Unregister For Events(event registration refnum=w374, error in=w373) -> (error out=w372:errorcluster)
            n127 = call <vilib>:"Add State(s) to Queue__jki_lib_state_machine.vi"("State(s) in (\"\")"=w377) -> ("States Out"=w376:string)  [unwired: 14 in]
          }
          frame "---------- Configuration ----------" {
            # "Do not put any code in this frame.\n(It is a separator no-op. You can make a copy of this frame to create a new UI frame)"
            n128 = call <vilib>:"Add State(s) to Queue__jki_lib_state_machine.vi"("State(s) in (\"\")"=w382) -> ("States Out"=w381:string)  [unwired: 14 in]
          }
          frame "Configuration: Initialize" {
            # "Do not put any code in this frame.\n(It is a separator no-op. You can make a copy of this frame to create a new UI frame)"
            n129 = Unbundle By Name(w390) -> ("Configuration"=w388:refnum<class "Configuration.lvclass">, "Instrument"=w389:refnum<class "Inst.AH2500.lvclass">)
            n130 = call <vilib>:"GetName.vi"("error in (no error)"=w392, "SMO"=w389) -> ("error out"=w391:errorcluster, "Name"=w393:string)  [unwired: 6 in, 2 out]
            n131 = call <userlib>:"Default Path.vi"("error in (no error)"=w391, "Folder Name [Application Name]"=w393, "Configuration in"=w388) -> ("error out"=w384:errorcluster, "Configuration out"=w387:refnum<class "Configuration.lvclass">)  [unwired: 7 in]
            n132 = call <userlib>:"Write Section.vi"("error in (no error)"=w384, "Section"="UI", "Configuration in"=w387) -> ("error out"=w383:errorcluster, "Configuration out"=w386:refnum<class "Configuration.lvclass">)  [unwired: 7 in]
            n133 = Bundle By Name(cluster=w390, "Configuration"=w386) -> (w394:T8)
            n134 = call <vilib>:"Add State(s) to Queue__jki_lib_state_machine.vi"("State(s) in (\"\")"=w397) -> ("States Out"=w396:string)  [unwired: 14 in]
          }
          frame "Configuration: Write UI Config File" {
            # "Do not put any code in this frame.\n(It is a separator no-op. You can make a copy of this frame to create a new Data frame)"
            n135 = Unbundle By Name(w402) -> ("Configuration"=w399:refnum<class "Configuration.lvclass">, "UI Cluster"=w401:T7)
            n136 = call <userlib>:"Write Configuration.vi"("error in (no error)"=w398, "Variant"=w401, "Configuration in"=w399) -> ("error out"=w400:errorcluster)  [unwired: 7 in, 1 out]
            n137 = call <vilib>:"Add State(s) to Queue__jki_lib_state_machine.vi"("State(s) in (\"\")"=w405) -> ("States Out"=w404:string)  [unwired: 14 in]
          }
          frame "Configuration: Read UI Config File" {
            # "Do not put any code in this frame.\n(It is a separator no-op. You can make a copy of this frame to create a new UI frame)"
            n138 = Unbundle By Name(w408) -> ("UI Cluster"=w411:T7, "Configuration"=w414:refnum<class "Configuration.lvclass">)
            n139 = call <userlib>:"Read Configuration.vi"("INI Fomatted Cluster Type"=w411, "error in (no error)"=w410, "Configuration in"=w414) -> ("error out"=w413:errorcluster, "Configuration"=w412:variant)  [unwired: 6 in, 1 out]
            n140 = Variant To Data(error in=w413, type=w411, Variant=w412) -> (data=w407:T7, error out=w409:errorcluster)
            n141 = Bundle By Name(cluster=w408, "UI Cluster"=w407) -> (w406:T8)
            n142 = call <vilib>:"Add State(s) to Queue__jki_lib_state_machine.vi"("State(s) in (\"\")"=w417) -> ("States Out"=w416:string)  [unwired: 14 in]
          }
          frame "---------- Action ----------" {
            n143 = Unbundle By Name(w419) -> ("Instrument"=w420:refnum<class "Inst.AH2500.lvclass">)
            n144 = Bundle By Name(cluster=w419, "Instrument"=w420) -> (w418:T8)
            n145 = call <vilib>:"Add State(s) to Queue__jki_lib_state_machine.vi"("State(s) in (\"\")"=w424) -> ("States Out"=w423:string)  [unwired: 14 in]
          }
          frame "Action: Notify UI Closed" {
            # "Notify that the UI has been closed"
            n146 = Unbundle By Name(w425) -> ("Instrument UI"=w428:refnum<class "Inst UI.AH2500.lvclass">)
            n147 = call <vilib>:"Hide.vi"("error in (no error)"=w427, "SMO.UI"=w428) -> ("error out"=w426:errorcluster)  [unwired: 8 in, 1 out]
            n148 = call <vilib>:"Add State(s) to Queue__jki_lib_state_machine.vi"("State(s) in (\"\")"=w431) -> ("States Out"=w430:string)  [unwired: 14 in]
          }
          frame "Action: getAll" {
            n149 = Unbundle By Name(w435) -> ("getAll"=w433:T6, "Instrument"=w438:refnum<class "Inst.AH2500.lvclass">)
            n150 = call "GET ALL.vim"("type"=w433, "error in (no error)"=w436, "Instrument in"=w438) -> ("error out"=w440:errorcluster, "getAll"=w432:T6, "Instrument out"=w434:refnum<class "Inst.AH2500.lvclass">)  [unwired: 6 in]
            n151 = Bundle By Name(cluster=w435, "Instrument"=w434, "getAll"=w432) -> (w437:T8)
            n152 = call <vilib>:"Add State(s) to Queue__jki_lib_state_machine.vi"("State(s) in Front (\"\")"="" ("State(s) in Front (\"\")"), "State(s) in (\"\")"=w443) -> ("States Out"=w442:string)  [unwired: 13 in]
          }
          frame "Action: Open" {
            n153 = Unbundle By Name(w450) -> ("Instrument"=w448:refnum<class "Inst.AH2500.lvclass">)
            n154 = call <userlib>:"Write Client Type.vi"("error in (no error)"=w445, "Client Type"=Client_Type--Enum."Local", "Instrument in"=w448) -> ("error out"=w446:errorcluster, "Instrument out"=w447:refnum<class "Inst.AH2500.lvclass">)  [unwired: 7 in]
            n155 = call-dynamic "Open.vi"("error in (no error)"=w446, "Inst.AH2500 in"=w447) -> ("error out"=w453:errorcluster, "Inst.AH2500 out"=w449:refnum<class "Inst.AH2500.lvclass">)  [unwired: 8 in]
            n156 = Bundle By Name(cluster=w450, "Instrument"=w449) -> (w451:T8)
            n157 = call <vilib>:"Add State(s) to Queue__jki_lib_state_machine.vi"("State(s) in Front (\"\")"="" ("State(s) in Front (\"\")"), "State(s) in (\"\")"=w456) -> ("States Out"=w455:string)  [unwired: 13 in]
          }
          frame "Action: Close" {
            n158 = Unbundle By Name(w458) -> ("Instrument"=w461:refnum<class "Inst.AH2500.lvclass">)
            n159 = call-dynamic "Close.vi"("error in (no error)"=w459, "Inst.AH2500 in"=w461) -> ("error out"=w463:errorcluster, "Inst.AH2500 out"=w457:refnum<class "Inst.AH2500.lvclass">)  [unwired: 8 in]
            n160 = Bundle By Name(cluster=w458, "Instrument"=w457) -> (w460:T8)
            n161 = call <vilib>:"Add State(s) to Queue__jki_lib_state_machine.vi"("State(s) in Front (\"\")"="" ("State(s) in Front (\"\")"), "State(s) in (\"\")"=w466) -> ("States Out"=w465:string)  [unwired: 13 in]
          }
          frame "Action: Send Message to Instrument" {
            # "Send a message (command, data, etc) to the Instrument:process.vi"
            n162 = Unbundle By Name(w471) -> ("Instrument"=w470:refnum<class "Inst.AH2500.lvclass">)  [unwired: 1 out]
            n163 = call <userlib>:"Instrument.MessageToProcess.vi"("error in (no error)"=w468, "Instrument"=w470) -> ("error out"=w467:errorcluster, "Instrument out"=w469:refnum<class "Inst.AH2500.lvclass">)  [unwired: 8 in]
            n164 = Bundle By Name(cluster=w471, "Instrument"=w469) -> (w472:T8)
            n165 = call <vilib>:"Add State(s) to Queue__jki_lib_state_machine.vi"("State(s) in Front (\"\")"="" ("State(s) in Front (\"\")"), "State(s) in (\"\")"=w476) -> ("States Out"=w475:string)  [unwired: 13 in]
          }
          frame "Action: Send Message to Child" {
            # "Send a message (command, data, etc) to the Instrument.Child:process.vi"
            n166 = Unbundle By Name(w481) -> ("Instrument"=w480:refnum<class "Inst.AH2500.lvclass">)  [unwired: 1 out]
            n167 = call "Inst.AH2500.MessageToProcess.vi"("error in (no error)"=w478, "Inst.AH2500 in"=w480) -> ("error out"=w477:errorcluster, "Inst.AH2500 out"=w479:refnum<class "Inst.AH2500.lvclass">)  [unwired: 8 in]
            n168 = Bundle By Name(cluster=w481, "Instrument"=w479) -> (w482:T8)
            n169 = call <vilib>:"Add State(s) to Queue__jki_lib_state_machine.vi"("State(s) in Front (\"\")"="" ("State(s) in Front (\"\")"), "State(s) in (\"\")"=w486) -> ("States Out"=w485:string)  [unwired: 13 in]
          }
        }
      }
    }
    frame Error {
    }
  }
  n170 = call-parent "Process.vi"("error in"=w5, "Instrument UI in"=w4) -> ("error out"=w2:errorcluster, "Instrument UI out"=→"Inst UI.AH2500 out":refnum<class "Inst UI.AH2500.lvclass">)  [unwired: 8 in]
  n171 = Merge Errors(w2, w1) -> (→"error out":errorcluster)
